vi "Handle.vi"(10 "log record":T1 {"timestamp" format="%<%x %.3X>T"}, 11 "direct handler in":refnum<class "Direct Handler.lvclass">) -> (0 "writer error":errorcluster, 1 "formatter error":errorcluster, 3 "direct handler out":refnum<class "Direct Handler.lvclass">)   [LabVIEW 2018, in "GLog.lvlib" / "Direct Handler.lvclass"]
uses:
  Direct Handler.lvclass
  Log Record.ctl
  logger_class/Internal Log Levels.ctl
  <vilib>/ErrorRing/Error Ring.xnode
  GLog.lvlib
panel:
  # "Connector Pane"
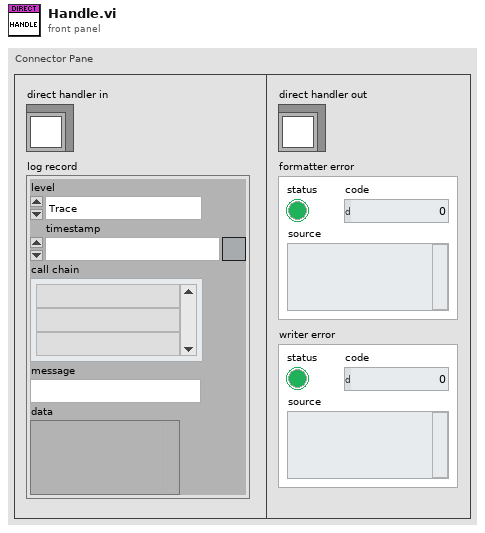
[diagram p1: front panel]
types:
  T1 = typedef "GLog.lvlib/Log Record.ctl" = cluster{"level":T2, "timestamp":timestamp, "call chain":string[], "message":string, "data":variant}
  T2 = typedef "GLog.lvlib/Internal Log Levels.ctl" = enum16{"Trace", "Debug", "Info", "Warning", "Error", "Critical", "Internal"}
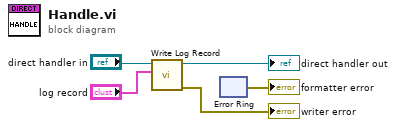
[diagram p0: block diagram]
diagram:
  n1 = call-dynamic "Write Log Record.vi"("log record"="log record", "direct handler in"="direct handler in") -> ("error out"=→"writer error":errorcluster, "direct handler out"=→"direct handler out":refnum<class "Direct Handler.lvclass">)  [unwired: 8 in]
  n2 = xnode "Error Ring"() -> ("error out"=→"formatter error":errorcluster)
